vi "Close output.vi"(7 "Original handle":u64, 8 "error in (no error)":errorcluster, 9 "Write handle":u64, 10 "Read handle":u64, 11 "STD IN/OUT":u32(ring)=4294967284 items=["STD_OUTPUT_HANDLE"=4294967285, "STD_ERROR_HANDLE"=4294967284]) -> (0 "error out":errorcluster)   [LabVIEW 2012, in "LightPipes.lvlib"]
uses:
  LightPipes.lvlib
  kernel32.dll
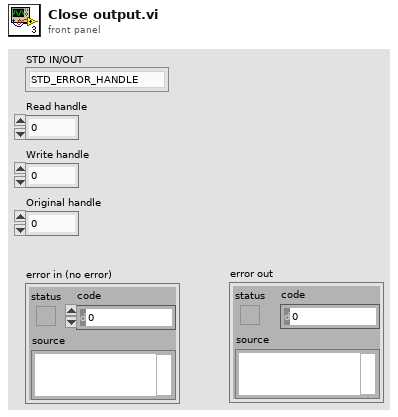
[diagram p1: front panel]
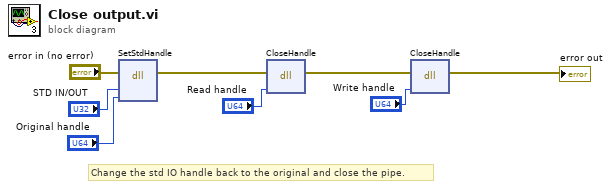
[diagram p0: block diagram]
diagram:
  # "Change the std IO handle back to the original and close the pipe."
  n1 = dll-call lib="kernel32.dll" fn="SetStdHandle"(error in="error in (no error)", "nStdHandle"="STD IN/OUT", "hHandle"="Original handle") -> (error out=w7:errorcluster)  [unwired: 5 in, 1 out]
  n2 = dll-call lib="kernel32.dll" fn="CloseHandle"(error in=w7, "hObject"="Read handle") -> (error out=w6:errorcluster)  [unwired: 4 in, 1 out]
  n3 = dll-call lib="kernel32.dll" fn="CloseHandle"(error in=w6, "hObject"="Write handle") -> (error out=→"error out":errorcluster)  [unwired: 4 in, 1 out]
